vi "Exercise1.13-State Indicator-S2.vi"() -> ()   [LabVIEW 2013]
panel:
  out "num":u32
  out "bool":bool[](array[boolean])
  out "Output2":dbl
  out "Output1":dbl
  in  "Input":dbl
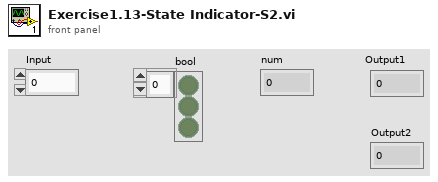
[diagram p1: front panel]
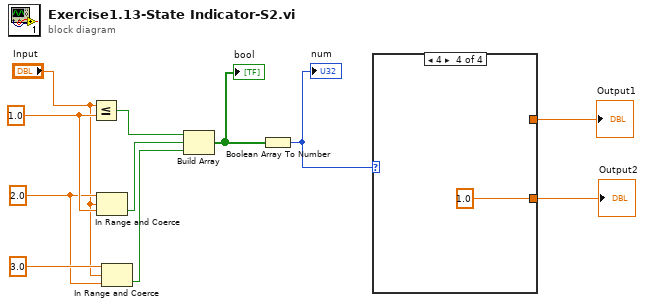
[diagram p0: block diagram]
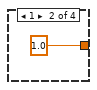
[diagram p3: hidden frame]
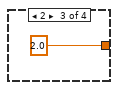
[diagram p4: hidden frame]
diagram:
  w9 = 2.0 ("上限")
  w11 = 1.0 ("y")
  n1 = Less Or Equal?(x="Input", y=w11) -> (x <= y?=w8:bool)
  n2 = In Range and Coerce(upper limit=w9, x="Input", lower limit=w11) -> (In Range?=w7:bool)  [unwired: 1 out]
  n3 = In Range and Coerce(upper limit=3.0 ("上限"), x="Input", lower limit=w9) -> (In Range?=w6:bool)  [unwired: 1 out]
  n4 = Build Array(w8, w7, w6) -> (w5:bool[])
  "bool" <- w5
  n5 = Boolean Array To Number(Boolean array=w5) -> (number=w3:u32)
  "num" <- w3
  n6 = case shown="4" w3 {
    tunnel: [_ 1.0 2.0 _] -> w2
    tunnel: [_ _ _ 1.0] -> w1
    frame 0, Default {
    }
    frame 1 {
    }
    frame 2 {
    }
    frame 4 {
    }
  }
  "Output1" <- w2
  "Output2" <- w1
